vi "Split Waveform for Transition Test.vi"(0 "Waveform In":waveform(dbl)={"t0"=timestamp(3433165898.5470004 s since 1904-01-01), "dt"=1e-05, "Y"=array[4250 elements]}, 5 "Final Threshold":dbl=2.5 format="%.2p", 7 "Samples before end":dbl=1000.0, 11 "error in (no error)":errorcluster) -> (4 "output waveform":waveform(dbl), 15 "error out":errorcluster)   [LabVIEW 2010]
uses:
  <vilib>/measure/mamon.llb/Trigger Detection for 1 Channel.vi
  <vilib>/Waveform/WDTOps.llb/WDT Get Waveform Subset DBL.vi
  <vilib>/measure/NI_MAPro.lvlib
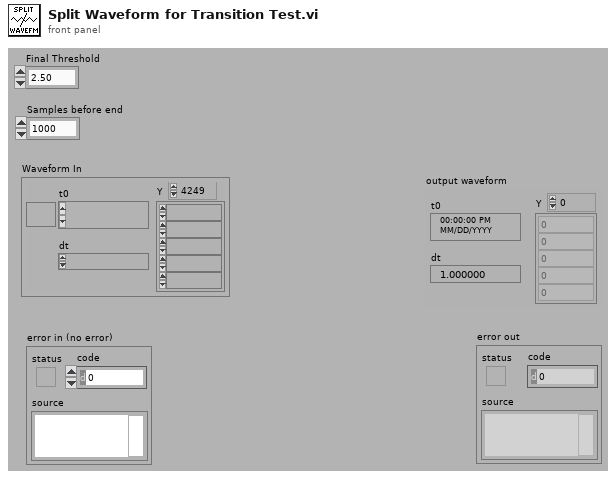
[diagram p1: front panel]
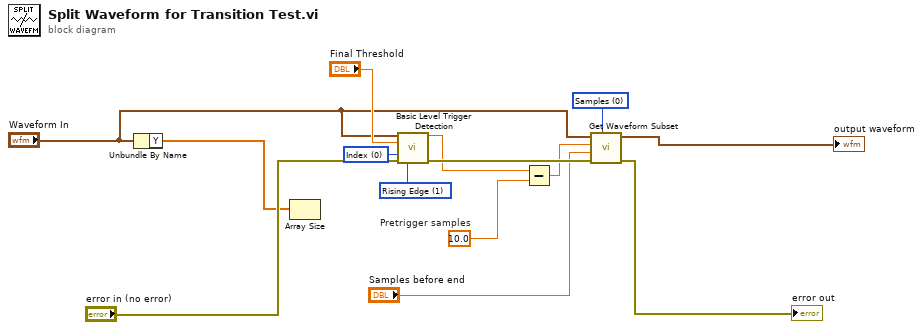
[diagram p0: block diagram]
diagram:
  w3 = 10.0  # Pretrigger samples
  w11 = u16 0 items=["Samples", "Relative Time"] ("start/duration format")
  w12 = u16 0 items=["Index", "Time"] ("location mode")
  w14 = u16 1 items=["Falling Edge", "Rising Edge"] ("trigger slope")
  n1 = Unbundle By Name("Waveform In") -> ("Y"=w7:dbl[])
  n2 = Array Size(array=w7) -> ()  [unwired: 1 out]
  n3 = call-poly <vilib>:"Basic Level Trigger Detection.vi"("signal in"="Waveform In", "level"="Final Threshold", "location mode"=w12, "error in (no error)"="error in (no error)", "trigger slope"=w14) -> ("trigger location"=w4:dbl, "error out"=w9:errorcluster)  [unwired: 8 in, 1 out]
  n4 = Subtract(x=w4, y=w3) -> (x-y=w2:dbl)
  n5 = call-poly <vilib>:"Get Waveform Subset.vi"("start/duration format"=w11, "error in (no error)"=w9, "duration"="Samples before end", "start samples/time"=w2, "waveform in"="Waveform In") -> ("error out"=→"error out":errorcluster, "waveform out"=→"output waveform":waveform(dbl))  [unwired: 1 in, 2 out]
